vi "XIPIN_VIO_(ChipScope_Pro_-_Virtual_Input_Output)_1_05_a.vi"   [LabVIEW 2017]
doc: "The Virtual Input/Output (VIO) core is a customizable core that can both monitor and drive internal FPGA signals in real time.\n------------------------------------\n<b>Need License</b> : No"
uses:
  <vilib>/rvi/XilinxIP/XIPIN_XNode/niFpgaXIPIN.xnode
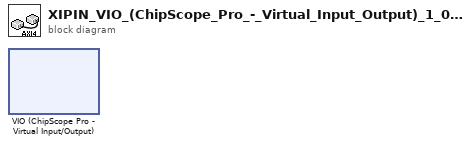
[diagram p0: block diagram]
diagram:
  n1 = xnode ("VIO (ChipScope Pro - Virtual Input/Output)")() -> ()
